vi "util_nearest_in_array.vi"(10 "desired element":dbl, 11 "1D Array":dbl[](array[numeric])) -> (0 "2nd closest index":i32, 1 "2nd closest element":dbl, 2 "closest index":i32, 3 "closest element":dbl)   [LabVIEW 2016]
panel:
  out "Altered array for finding 2nd closest":dbl[](array[numeric])
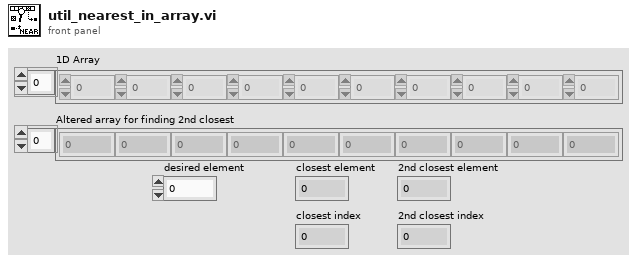
[diagram p1: front panel]
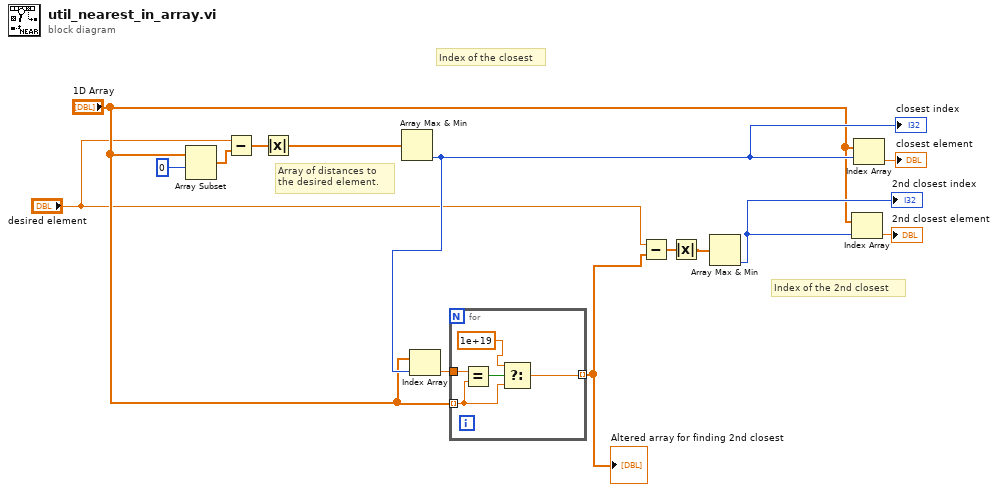
[diagram p0: block diagram]
diagram:
  # "Index of the 2nd closest"
  # "Index of the closest"
  # "Array of distances to the desired element."
  n1 = Array Subset(array="1D Array", index=0) -> (w12:dbl[])  [unwired: 1 in]
  n2 = Subtract(x="desired element", y=w12) -> (x-y=w14:dbl[])
  n3 = Absolute Value(x=w14) -> (abs(x)=w8:dbl[])
  n4 = Array Max & Min(array=w8) -> (min index (indices)=w7:i32)  [unwired: 3 out]
  "closest index" <- w7
  n5 = Index Array(array="1D Array", index=w7) -> (element=w6:dbl)
  n6 = for {
    tunnel: "1D Array" -> [w16] mode=indexing
    tunnel: w6 -> [w19]
    tunnel: [w15] -> w2 mode=indexing
    n7 = Equal?(x=w19, y=w16) -> (x = y?=w18:bool)
    n8 = Select(t=1e+19 ("new element/subarray"), s=w18, f=w16) -> (s? t:f=w15:dbl)
  }
  "Altered array for finding 2nd closest" <- w2
  n9 = Subtract(x="desired element", y=w2) -> (x-y=w3:dbl[])
  n10 = Absolute Value(x=w3) -> (abs(x)=w4:dbl[])
  n11 = Array Max & Min(array=w4) -> (min index (indices)=w9:i32)  [unwired: 3 out]
  "2nd closest index" <- w9
  n12 = Index Array(array="1D Array", index=w9) -> (element=→"2nd closest element":dbl)
  n13 = Index Array(array="1D Array", index=w7) -> (element=→"closest element":dbl)
